vi "makeNames_remove underscores.vi"(11 "Strings":string[](array[string])) -> (3 "Names":string[](array[string]))   [LabVIEW 2021]
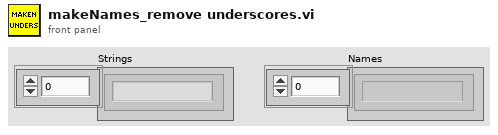
[diagram p1: front panel]
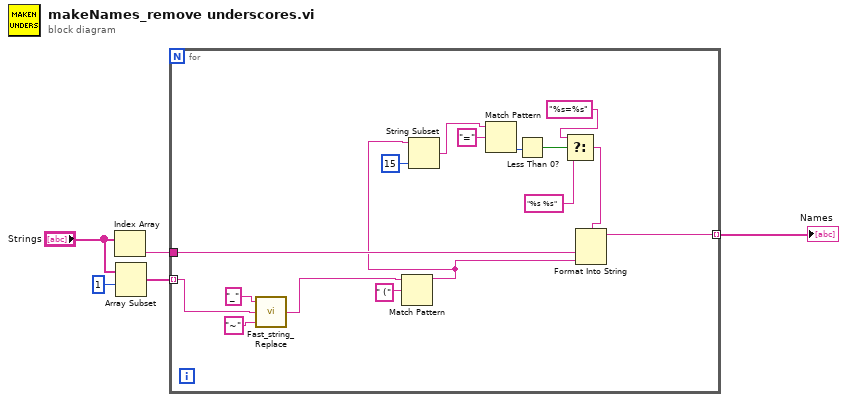
[diagram p0: block diagram]
diagram:
  n1 = Index Array(array="Strings") -> (element=w1:string)  [unwired: 1 in]
  n2 = Array Subset(array="Strings", index=1) -> (w2:string[])  [unwired: 1 in]
  n3 = for {
    tunnel: w2 -> [w7] mode=indexing
    tunnel: [w19] -> w4 mode=indexing
    tunnel: w1 -> [w20]
    n4 = call "Fast_string_Replace.vi"("Replace match with:"="~", "Input String"=w7, "regular expression"="_") -> ("Output String"=w6:string)  [unwired: 2 out]
    n5 = Match Pattern(string=w6, regular expression=" (") -> (before substring=w15:string)  [unwired: 4 out]
    n6 = String Subset(string=w15, length (rest)=15 ("length (rest)")) -> (substring=w14:string)  [unwired: 1 in]
    n7 = Match Pattern(string=w14, regular expression="=") -> (offset past match=w17:i32)  [unwired: 1 in, 3 out]
    n8 = Less Than 0?(x=w17) -> (x < 0?=w13:bool)
    n9 = Select(t="%s=%s" ("format string"), s=w13, f="%s %s" ("Format String")) -> (s? t:f=w11:string)
    n10 = Format Into String(format string=w11, w20, w15) -> (resulting string=w19:string)  [unwired: 2 in, 1 out]
  }
  "Names" <- w4
